vi "modbusIRQTriggerLoop.vi"(11 "Modbus Port Settings":T1={"Tx Port"="ModbusPort1Tx", "Tx Data FIFO"="txModbusPort1FIFO", "Tx Internal FIFO"="txModbusPort1InternalFIFO", "Tx Telemetry FIFO"="txModbusPort1TelemetryFIFO", "Rx Port"="ModbusPort1Rx", "Rx Data FIFO"="rxModbusPort1FIFO", "Rx Telemetry FIFO"="txModbusPort1TelemetryFIFO", "Base Telemetry Address"=0, "Wait For Rx Frame Register"="WaitForPort1RxFrame", "IRQ Address"=0, "Trigger IRQ Register"="TriggerPort1IRQ", "Trigger IRQ Response Register"="TriggerPort1IRQ"}) -> ()   [LabVIEW 2015]
uses:
  DataTypes/ModbusPortSettings.ctl
  <vilib>/rvi/Emulation/niFpgaGetClockAttributes.vi
  <vilib>/rvi/Emulation/niFpgaSctlEmulationGetInTimedLoop.vi
  <vilib>/rvi/Emulation/niFpgaEmulationReportErrorSimple.vi
  <vilib>/rvi/Emulation/niFpgaEmulationIsFPGAContextNoSignature.vi
  <vilib>/rvi/DataTransferAndStorage/Container/Common/niFpgaContainerGetUniqueNameForEmu.vi
  <vilib>/rvi/Memory/Memory_Emulation/niFpgaMemoryEmulationCacheClearOnFirstRun.vi
  <vilib>/rvi/Memory/Memory_Emulation/nirvimemoryEmulationManagerCache_MakeExclusive.vi
  <vilib>/rvi/Memory/Memory_Emulation/niFpgaMemoryEmulationValidateCache.vi
  <vilib>/rvi/Memory/Memory_Emulation/nirvimemoryEmulationManagerCache_InsertValue.vi
  <vilib>/Utility/error.llb/Clear Errors.vi
  <vilib>/rvi/Memory/Memory_Emulation/nirvimemoryEmulationManagerCache_ReleaseExclusive.vi
  <vilib>/rvi/Memory/Memory_Emulation/nirvimemoryEmulationManagerCache_GetValue.vi
  <vilib>/rvi/Memory/Memory_Emulation/nirvimemoryEmulationManagerCache_SetValue.vi
  <vilib>/rvi/Emulation/niFpgaProcessEmulError.vi
  <vilib>/rvi/DataTransferAndStorage/Container/Common/niFpgaContainerExecOnDevCompGetState.vi
  <vilib>/rvi/Emulation/niFpgaCriticalErrorInLSC.vi
  <vilib>/rvi/DataTransferAndStorage/Container/XNode/niFpgaContainer.xnode
  <vilib>/rvi/DataTransferAndStorage/Register/Emulation/niFpgaRegisterEmulation.vi
  <vilib>/rvi/DataTransferAndStorage/Register/Emulation/niFpgaRegisterEmulationRefIn.vi
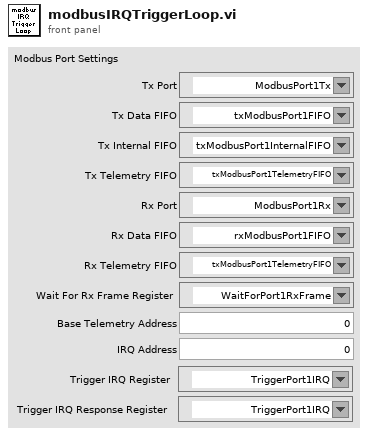
[diagram p1: front panel]
types:
  T1 = typedef "ModbusPortSettings.ctl" = cluster{"Tx Port":refnum<k21>, "Tx Data FIFO":refnum<k21>, "Tx Internal FIFO":refnum<k21>, "Tx Telemetry FIFO":refnum<k21>, "Rx Port":refnum<k21>, "Rx Data FIFO":refnum<k21>, "Rx Telemetry FIFO":refnum<k21>, "Base Telemetry Address":u32, "Wait For Rx Frame Register":refnum<k21>, "IRQ Address":u8, "Trigger IRQ Register":refnum<k21>, "Trigger IRQ Response Register":refnum<k21>}
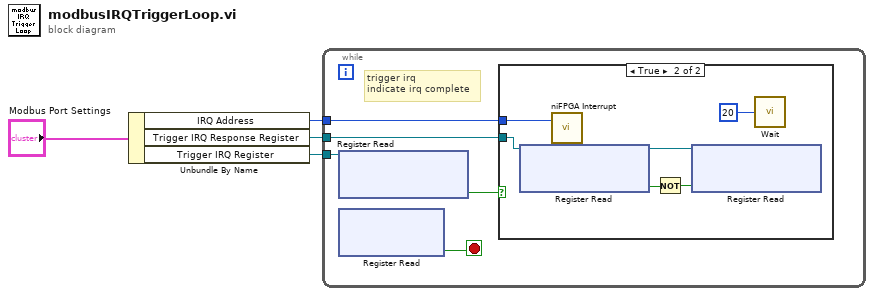
[diagram p0: block diagram]
diagram:
  n1 = Unbundle By Name("Modbus Port Settings") -> ("IRQ Address"=w2:u8, "Trigger IRQ Response Register"=w4:refnum<k21>, "Trigger IRQ Register"=w3:refnum<k21>)
  n2 = while {
    tunnel: w2 -> [w6]
    tunnel: w3 -> [w8]
    tunnel: w4 -> [w5]
    stop <- w9 stop-if-true
    # "trigger irq\nindicate irq complete"
    n3 = xnode ("Register Read")("Register In"=w8) -> ("Data"=w7:bool)  [unwired: 1 out]
    n4 = xnode ("Register Read")() -> ("Data"=w9:bool)  [unwired: 1 in, 1 out]
    n5 = case shown="True" w7 {
      tunnel: w6 -> [_ w15]
      tunnel: w5 -> [_ w13]
      frame False {
      }
      frame True {
        n6 = xnode ("Register Read")("Register In"=w13) -> ("Data"=w12:bool, "Register Out"=w14:refnum<k21>)
        n7 = call <vilib>:"niFPGA Interrupt.vi"("IRQ Number (0)"=w15) -> ()  [unwired: 2 in]
        n8 = Not(x=w12) -> (.not. x?=w11:bool)
        n9 = xnode ("Register Read")("Data"=w11, "Register In"=w14) -> ()  [unwired: 1 out]
        n10 = call "Wait"("Count(Ticks)"=u32 20) -> ()  [unwired: 1 out]
      }
    }
  }
